vi "MSEncoder Case-1-Start.vi"(8 "error in (no error)":errorcluster, 9 "ParamValIn":variant, 11 "MSEncoder in":refnum<class "MSEncoder.lvclass">) -> (0 "error out":errorcluster, 1 "Msg":string, 3 "MSEncoder out":refnum<class "MSEncoder.lvclass">)   [LabVIEW 2018, in "MSEncoder.lvclass"]
uses:
  MSEncoder.lvclass
  Ctl/MSEditorParam RFStart.ctl
  PublicSubVI/Ctl/MathieuEqParam.ctl
  MSEncoder.lvclass/MSEncoder.ctl
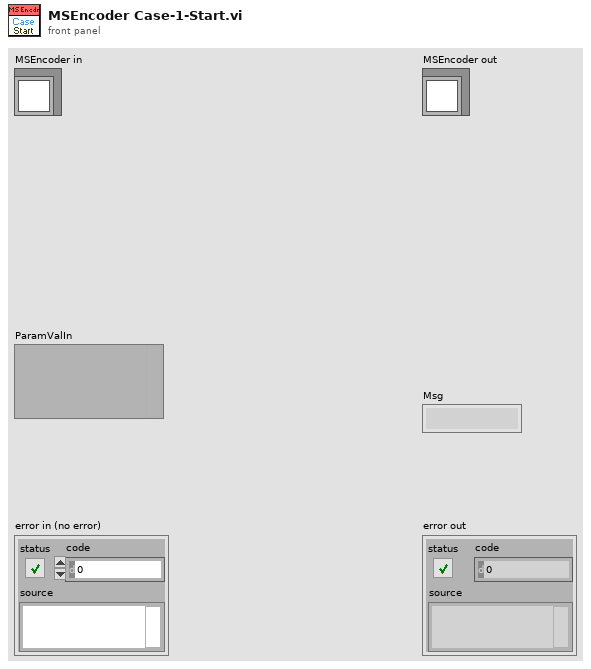
[diagram p1: front panel]
types:
  T1 = typedef "MSEditorParam RFStart.ctl" = cluster{"freq":ext, "amp":ext, "wfmType":u32}
  T2 = typedef "MathieuEqParam.ctl" = cluster{"mz(Th)":ext, "Amp(V)":ext, "Freq(Hz)":ext, "Beta":ext, "r_0 (mm)":ext, "z_0 (mm)":ext}
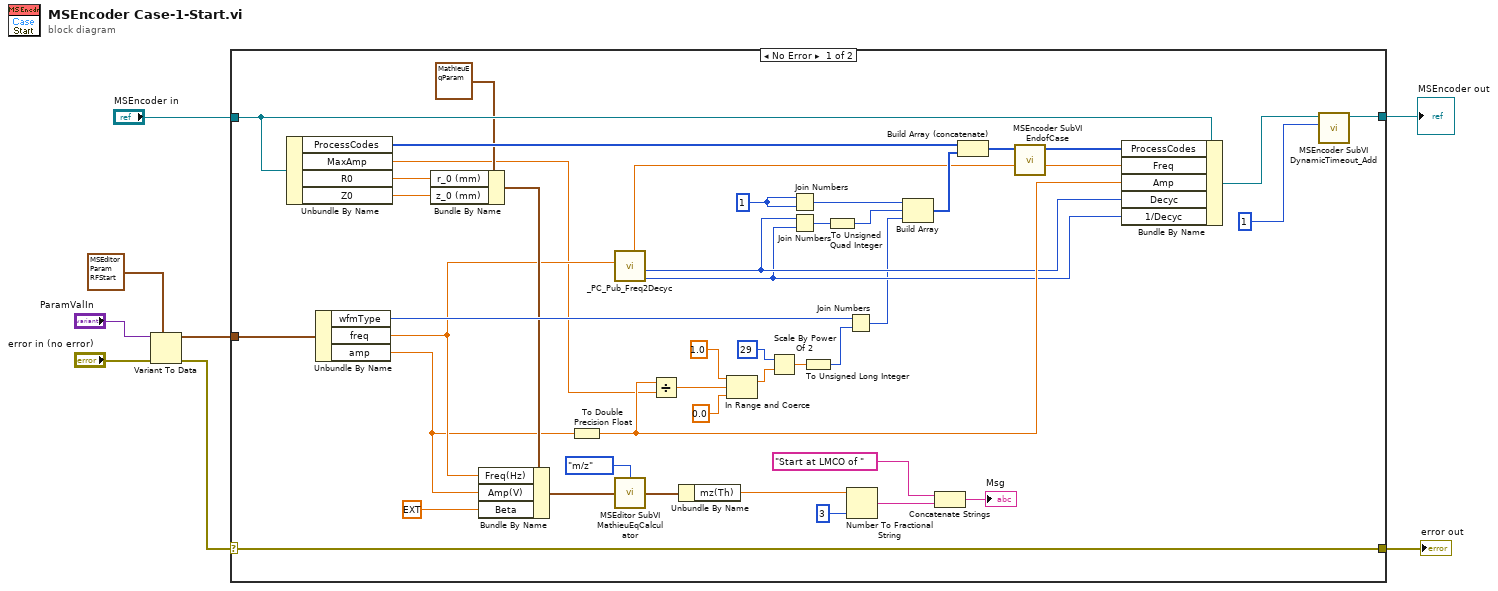
[diagram p0: block diagram]
diagram:
  n1 = Variant To Data(error in="error in (no error)", type=T1 {"freq"=0.001, "amp"=0.01, "wfmType"=0} ("ParamValueType"), Variant="ParamValIn") -> (data=w4:T1, error out=w2:errorcluster)
  n2 = case shown="No Error" w2 {
    selector: w2 -> [w51 w53]
    tunnel: "MSEncoder in" -> [w50 w52]
    tunnel: [w51 w53] -> w1
    tunnel: [w26 w52] -> w7
    tunnel: w4 -> [w49 _]
    frame No Error {
      w41 = u32 1
      n3 = Unbundle By Name(w50) -> ("ProcessCodes"=w33:u64[], "MaxAmp"=w9:dbl, "R0"=w23:ext, "Z0"=w22:ext)
      n4 = Unbundle By Name(w49) -> ("wfmType"=w29:u32, "freq"=w20:ext, "amp"=w19:ext)
      n5 = Bundle By Name(cluster=T2 {"mz(Th)"=0.0, "Amp(V)"=330.0, "Freq(Hz)"=0.0, "Beta"=1.0, "r_0 (mm)"=10.0, "z_0 (mm)"=7.0710678118654755} ("Parametres in"), "r_0 (mm)"=w23, "z_0 (mm)"=w22) -> (w21:T2)
      n6 = Bundle By Name(cluster=w21, "Freq(Hz)"=w20, "Amp(V)"=w19, "Beta"=ext 1.0) -> (w18:T2)
      n7 = To Double Precision Float(number=w19) -> (double precision float=w37:dbl)
      n8 = call "_PC_Pub_Freq2Decyc.vi"("Freq"=w20) -> ("(1/Decyc)*2^8"=w35:u32, "Decyc*2^32"=w36:u32, "Actual Freq"=w31:dbl)  [unwired: 4 in, 2 out]
      n9 = call "MSEditor SubVI MathieuEqCalculator.vi"("Target (Freq)"=enum16{"m/z", "Volt", "Freq", "Beta"}."m/z", "Parametres in"=w18) -> ("Parametres out"=w15:T2)  [unwired: 2 in]
      n10 = Divide(x=w37, y=w9) -> (x/y=w48:dbl)
      n11 = Unbundle By Name(w15) -> ("mz(Th)"=w14:ext)
      n12 = In Range and Coerce(upper limit=1.0, x=w48, lower limit=0.0) -> (coerced(x)=w45:dbl)  [unwired: 1 out]
      n13 = Scale By Power Of 2(n=i16 29, x=w45) -> (x*2^n=w43:dbl)
      n14 = Join Numbers(hi=w41, lo=w41) -> ((hi.lo)=w39:u64)
      n15 = Join Numbers(hi=w36, lo=w35) -> ((hi.lo)=w42:u64)
      n16 = To Unsigned Long Integer(number=w43) -> (unsigned 32bit integer=w30:u32)
      n17 = To Unsigned Quad Integer(1:w42) -> (0:w40:u64)
      n18 = Join Numbers(hi=w29, lo=w30) -> ((hi.lo)=w28:u64)
      n19 = Number To Fractional String(number=w14, precision (6)=i16 3) -> (F-format string=w11:string)  [unwired: 2 in]
      n20 = Build Array(w39, w40, w28) -> (w38:u64[])
      n21 = Concatenate Strings("Start at LMCO of ", w11) -> (→"Msg":string)
      n22 = Build Array (concatenate)(w33, w38) -> (w34:u64[])
      n23 = call "MSEncoder SubVI EndofCase.vi"("Case codes"=w34) -> ("Case codes with end"=w32:u64[])  [unwired: 9 in, 1 out]
      n24 = Bundle By Name(cluster=w50, "ProcessCodes"=w32, "Freq"=w31, "Amp"=w37, "Decyc"=w36, "1/Decyc"=w35) -> (w27:refnum<class "MSEncoder.lvclass">)
      n25 = call "MSEncoder SubVI DynamicTimeout_Add.vi"("Timeout_ms"=1, "MSEncoder"=w27) -> ("MSEncoder"=w26:refnum<class "MSEncoder.lvclass">)  [unwired: 8 in, 1 out]
    }
    frame Error {
    }
  }
  "error out" <- w1
  "MSEncoder out" <- w7
